vi "FGV_GPIB_Interface.vi"(2 "GPIB_Interface_In":string, 3 "Operation":enum16{"Get", "Set"}(ring)) -> (0 "GPIB_Interface_Out":string)   [LabVIEW 2014]
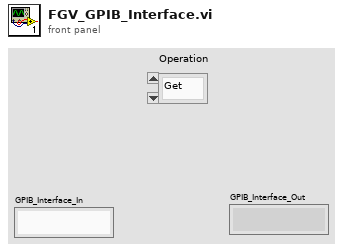
[diagram p1: front panel]
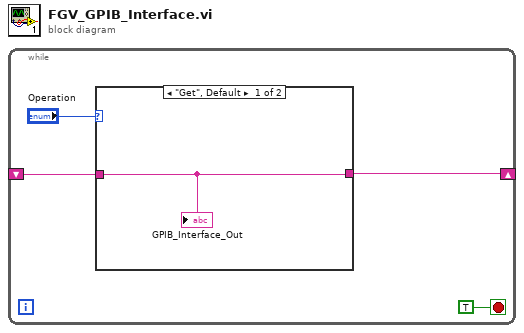
[diagram p0: block diagram]
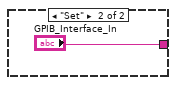
[diagram p2: hidden frame]
diagram:
  n1 = while {
    shift-right: [w2] -> _
    shift-left: _ -> [w1]
    stop <- TRUE stop-if-true
    n2 = case shown="\"Get\", Default" "Operation" {
      tunnel: [w5 "GPIB_Interface_In"] -> w2
      tunnel: w1 -> [w5 _]
      frame "Get", Default {
        "GPIB_Interface_Out" <- w5
      }
      frame "Set" {
      }
    }
  }
